vi "CRC16校验_string.vi"(10 "输入数据":string) -> (1 "高字节":u8 format="%x", 3 "低字节":u8 format="%x")   [LabVIEW 2010]
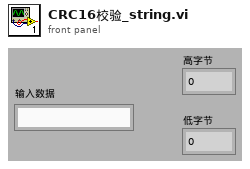
[diagram p1: front panel]
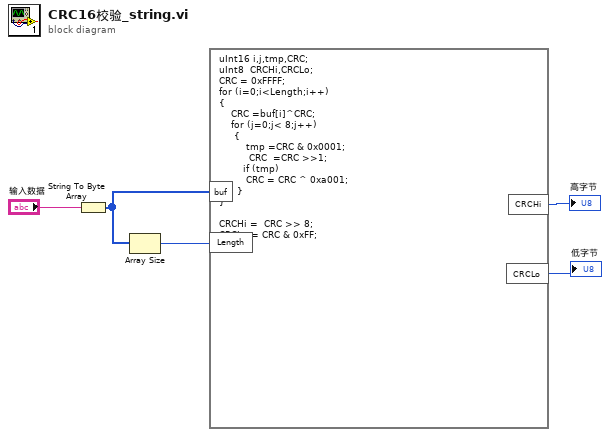
[diagram p0: block diagram]
diagram:
  n1 = String To Byte Array(string="输入数据") -> (unsigned byte array=w2:u8[])
  n2 = Array Size(array=w2) -> (size(s)=w3:i32)
  n3 = formula code="uInt16 i,j,tmp,CRC;\nuInt8  CRCHi,CRCLo;\nCRC = 0xFFFF;\nfor (i=0;i<Length;i++)\n{\n    CRC =buf[i]^CRC;\n    for (j=0;j< 8;j++)\n     {\n         tmp =CRC & 0x0001;\n          CRC  =CRC >>1;\n        if (tmp)\n         CRC = CRC ^ 0xa001;    \n      }\n}\n\nCRCHi =  CRC >> 8;\nCRCLo = CRC & 0xFF;"("buf"=w2, "Length"=w3) -> ("CRCLo"=→"低字节":u8, "CRCHi"=→"高字节":u8)
